vi "Open.vi"(8 "Error In":errorcluster, 10 "SSD1306 Channels":T1, 11 "LINX Resource":T2) -> (0 "Error Out":errorcluster, 3 "LINX Resource":T2)   [LabVIEW 2011, in "LVH-LINX.lvlib" / "SSD1306.lvlib"]
doc: "Power up the SSD1306 and bring it out of reset."
uses:
  SSD1306.lvlib
  Private/Type Defs/LINX Ref.ctl
  Private/Type Defs/Platform.ctl
  Private/Type Defs/Interface.ctl
  Private/Device/Type Defs/LINX Device Config.ctl
  Private/Device/Type Defs/TCP Config.ctl
  Private/Type Defs/Device Family.ctl
  Private/SSD1306 Config.ctl
  Private/SSD1306 FGV State.ctl
  Peripherals/Digital/Digital Write N Chans.vi
  Peripherals/Digital/Digital Write 1 Chan.vi
  LVH-LINX.lvlib
  Private/Device/Device.lvlib
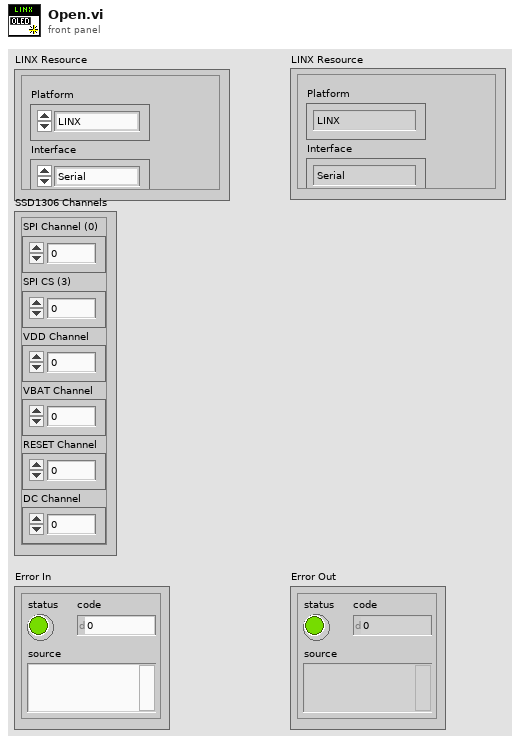
[diagram p1: front panel]
types:
  T1 = typedef "LVH-LINX.lvlib/SSD1306.lvlib/SSD1306 Config.ctl" = cluster{"SPI Channel (0)":u8, "VDD Channel":u8, "VBAT Channel":u8, "RESET Channel":u8, "DC Channel":u8, "SPI CS (3)":u8}
  T2 = typedef "LVH-LINX.lvlib/LINX Ref.ctl" = cluster{"Platform":T3, "Interface":T4, "LINX Device Config":T5}
  T3 = typedef "LVH-LINX.lvlib/Platform.ctl" = enum16{"LINX", "myRIO"}
  T4 = typedef "LVH-LINX.lvlib/Interface.ctl" = enum16{"Serial", "TCP"}
  T5 = typedef "LVH-LINX.lvlib/Device.lvlib/LINX Device Config.ctl" = cluster{"Interface":T4, "COM Port":refnum<visa-resource-name>, "TCP Configuration":T6, "Device Family":T7, "Device ID":u8, "Device Name":string, "TCP Ref":refnum<k5>}
  T6 = typedef "LVH-LINX.lvlib/Device.lvlib/TCP Config.ctl" = cluster{"IP Address":string, "Port":u16}
  T7 = typedef "LVH-LINX.lvlib/Device Family.ctl" = enum8{"National Instruments", "Digilent", "Arduino"}
  T8 = typedef "LVH-LINX.lvlib/SSD1306.lvlib/SSD1306 FGV State.ctl" = enum16{"Init", "Set", "Get"}
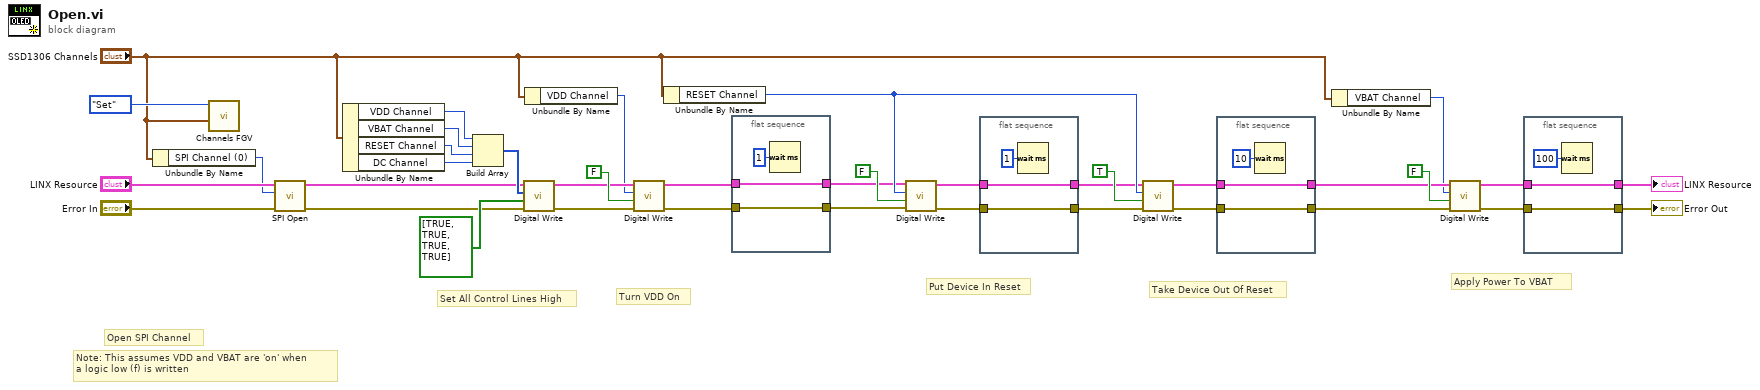
[diagram p0: block diagram]
diagram:
  # "Apply Power To VBAT"
  # "Take Device Out Of Reset"
  # "Put Device In Reset"
  # "Turn VDD On"
  # "Note: This assumes VDD and VBAT are 'on' when \na logic low (f) is written"
  # "Set All Control Lines High"
  # "Open SPI Channel"
  n1 = Unbundle By Name("SSD1306 Channels") -> ("SPI Channel (0)"=w3:u8)
  n2 = call "Channels FGV.vi"("SSD1306 Channels"="SSD1306 Channels", "SSD1306 FGV State"=SSD1306_FGV_State."Set") -> ()  [unwired: 9 in, 1 out]
  n3 = call "SPI Open.vi"("Error In"="Error In", "SPI Channel (0)"=w3, "LINX Resource"="LINX Resource") -> ("Error Out"=w1:errorcluster, "LINX Resource"=w2:T2)  [unwired: 7 in]
  n4 = Unbundle By Name("SSD1306 Channels") -> ("VDD Channel"=w29:u8, "VBAT Channel"=w35:u8, "RESET Channel"=w34:u8, "DC Channel"=w33:u8)
  n5 = Build Array(w29, w35, w34, w33) -> (w32:u8[])
  n6 = call-poly "Digital Write.vi"("Error In"=w1, "Values"=bool[] [TRUE, TRUE, TRUE, TRUE], "DO Channels"=w32, "LINX Resource"=w2) -> ("Error Out"=w30:errorcluster, "LINX Resource"=w27:T2)  [unwired: 6 in]
  n7 = Unbundle By Name("SSD1306 Channels") -> ("VDD Channel"=w25:u8)
  n8 = call-poly "Digital Write.vi"("Error In"=w30, "Output Value"=FALSE, "DO Channel"=w25, "LINX Resource"=w27) -> ("Error Out"=w7:errorcluster, "LINX Resource"=w6:T2)  [unwired: 6 in]
  n9 = Unbundle By Name("SSD1306 Channels") -> ("RESET Channel"=w19:u8)
  n10 = flat-sequence {
    tunnel: w7 -> [w40]
    tunnel: w6 -> [w39]
    tunnel: [w40] -> w5
    tunnel: [w39] -> w4
    frame #0 {
      n11 = Wait (ms)(milliseconds to wait=u32 1) -> ()  [unwired: 1 out]
    }
  }
  n12 = call-poly "Digital Write.vi"("Error In"=w5, "Output Value"=FALSE, "DO Channel"=w19, "LINX Resource"=w4) -> ("Error Out"=w24:errorcluster, "LINX Resource"=w23:T2)  [unwired: 6 in]
  n13 = flat-sequence {
    tunnel: w24 -> [w43]
    tunnel: w23 -> [w42]
    tunnel: [w43] -> w17
    tunnel: [w42] -> w18
    frame #0 {
      n14 = Wait (ms)(milliseconds to wait=u32 1) -> ()  [unwired: 1 out]
    }
  }
  n15 = call-poly "Digital Write.vi"("Error In"=w17, "Output Value"=TRUE, "DO Channel"=w19, "LINX Resource"=w18) -> ("Error Out"=w21:errorcluster, "LINX Resource"=w22:T2)  [unwired: 6 in]
  n16 = flat-sequence {
    tunnel: w21 -> [w46]
    tunnel: w22 -> [w45]
    tunnel: [w46] -> w12
    tunnel: [w45] -> w13
    frame #0 {
      n17 = Wait (ms)(milliseconds to wait=u32 10) -> ()  [unwired: 1 out]
    }
  }
  n18 = Unbundle By Name("SSD1306 Channels") -> ("VBAT Channel"=w10:u8)
  n19 = call-poly "Digital Write.vi"("Error In"=w12, "Output Value"=FALSE, "DO Channel"=w10, "LINX Resource"=w13) -> ("Error Out"=w15:errorcluster, "LINX Resource"=w14:T2)  [unwired: 6 in]
  n20 = flat-sequence {
    tunnel: w15 -> [w49]
    tunnel: w14 -> [w48]
    tunnel: [w49] -> w9
    tunnel: [w48] -> w8
    frame #0 {
      n21 = Wait (ms)(milliseconds to wait=u32 100) -> ()  [unwired: 1 out]
    }
  }
  "Error Out" <- w9
  "LINX Resource" <- w8
